vi "Project g.vi"() -> ()   [LabVIEW 2023]
uses:
  <vilib>/DAQmx/read.llb/DAQmx Read (Analog 1D DBL 1Chan NSamp).vi
  <vilib>/Analysis/baseanly.llb/Mean (DBL).vi
  <vilib>/DAQmx/create/channels.llb/DAQmx Create Channel (AI-Voltage-Basic).vi
  <vilib>/DAQmx/configure/timing.llb/DAQmx Timing (Sample Clock).vi
  <vilib>/DAQmx/configure/trigger.llb/DAQmx Start Trigger (Analog Edge).vi
  <vilib>/DAQmx/miscellaneous.llb/DAQmx Fill In Error Info.vi
  <vilib>/Analysis/NI_AALBase.lvlib
panel:
  in  "Elevation (m)":dbl
  in  "Latitude (rad)":dbl
  out "Experimental Acceleration (m/s²)":dbl
  out "Percent Error":dbl
  out "Theoretical Local Gravity Acceleration (m/s²)":dbl
  out "?":bool
  in  "File operation":T1(ring)=enum."open or create"
  in  "Select a file to save to":path
  out "Acceleration vs. Time":cluster{dbl[], "dX/dt":dbl[]}(graph)
  in  "Triggering system":bool
  in  "Sample mode":i32(ring)=10178 items=["Finite Samples"=10178, "Continuous Samples"=10123, "Hardware Timed Single Point"=12522]
  in  "# Samples":i32=1000
  in  "DAQ Rate":dbl=5000.0
  out "Displacement vs. Time":cluster{dbl[], dbl[]}(graph)
  in  "stop":bool
  in  "# Loops \n(For continuous samples)":i32
  in  "Custom scale name":tag="LaserDicplacement (mm)(ST06)(Monday)"
  in  "Physical channels":tag="cDAQ2Mod1/ai0"
  # "DAQ Input"
  # "File information"
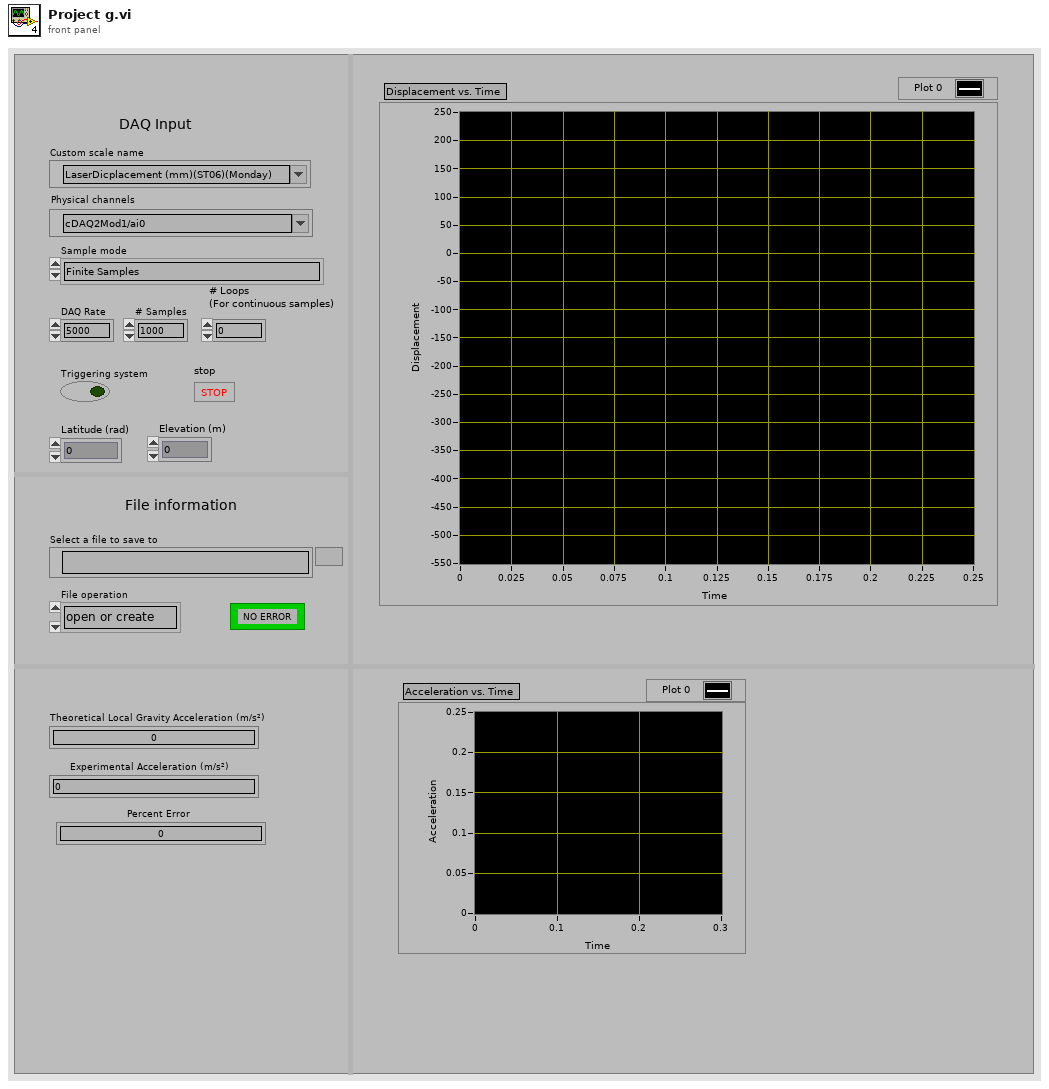
[diagram p1: front panel]
types:
  T1 = enum16{"open", "replace", "create", "open or create", "replace or create", "replace or create with confirmation"}
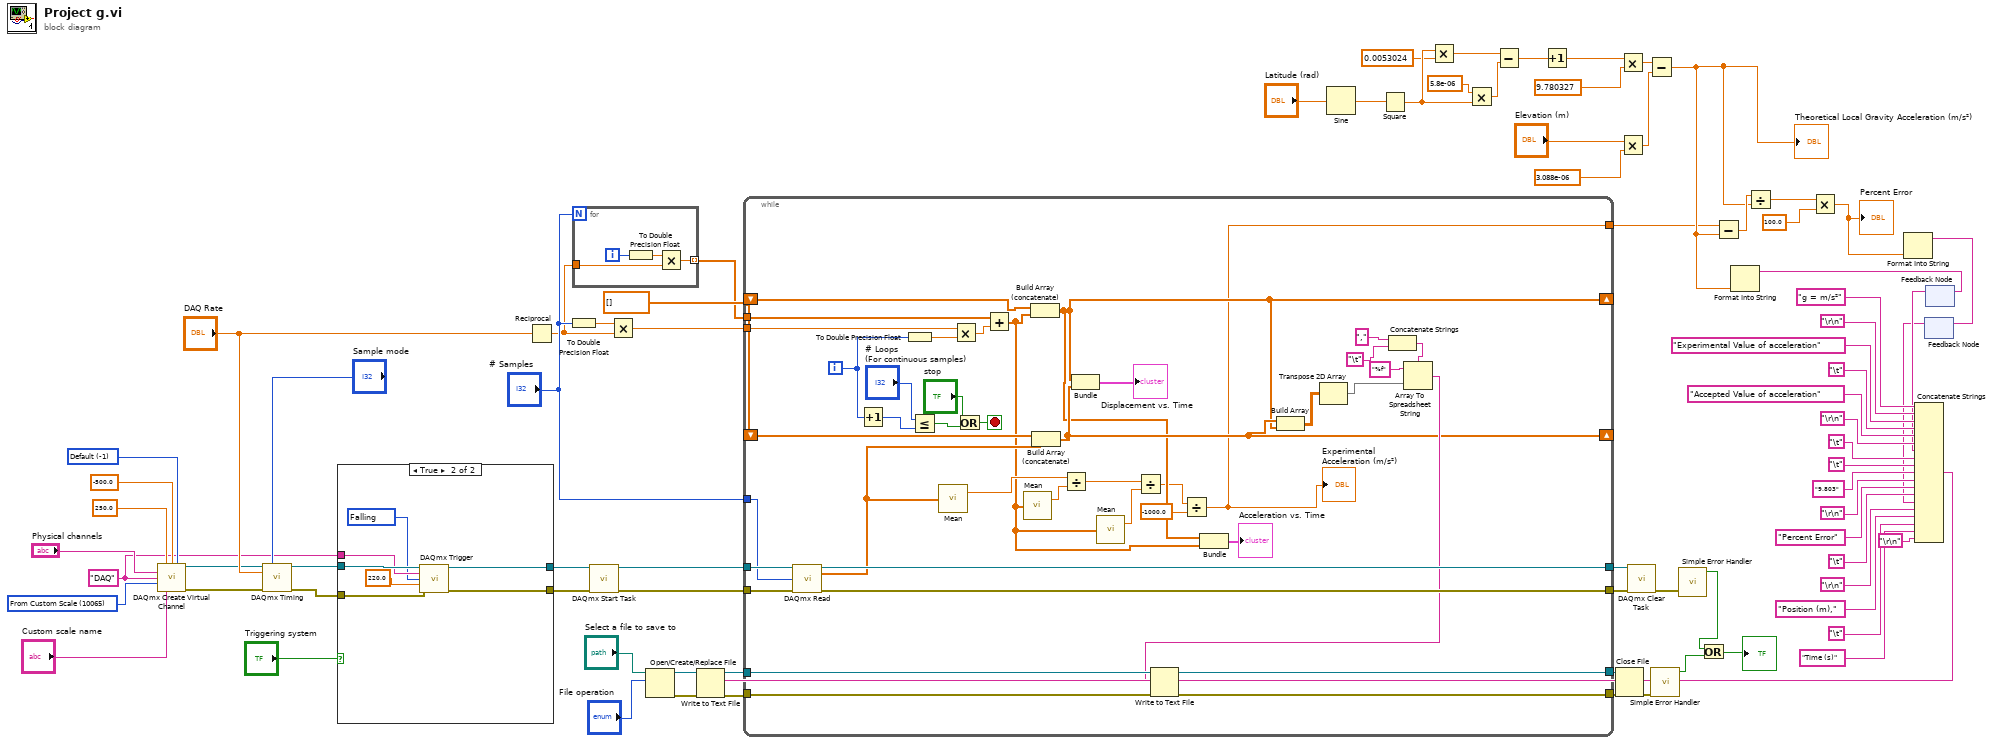
[diagram p0: block diagram]
diagram:
  w57 = "DAQ" ("name to assign")
  w71 = dbl[] []
  w76 = 10065 items=["Volts"=10348, "From Custom Scale"=10065] ("units")
  w79 = -1 items=["Default"=-1, "RSE"=10083, "NRSE"=10078, "Differential"=10106, "Pseudodifferential"=12529] ("input terminal configuration")
  n1 = call-poly <vilib>:"DAQmx Create Virtual Channel.vi"("maximum value"=250.0, "minimum value"=-500.0, "input terminal configuration"=w79, "physical channels"="Physical channels", "name to assign"=w57, "units"=w76, "custom scale name"="Custom scale name") -> ("task out"=w64:refnum<k21>, "error out"=w63:errorcluster)  [unwired: 7 in]
  n2 = call-poly <vilib>:"DAQmx Timing.vi"("task/channels in"=w64, "sample mode"="Sample mode", "rate"="DAQ Rate", "error in"=w63) -> ("task out"=w60:refnum<k21>, "error out"=w59:errorcluster)  [unwired: 10 in]
  n3 = case shown="True" "Triggering system" {
    tunnel: [w83 w86] -> w62
    tunnel: [w82 w85] -> w61
    tunnel: w60 -> [w83 w89]
    tunnel: w59 -> [w82 w88]
    tunnel: w57 -> [_ w87]
    frame False {
    }
    frame True {
      w84 = 10171 items=["Rising"=10280, "Falling"=10171] ("slope")
      n4 = call-poly <vilib>:"DAQmx Trigger.vi"("task/channels in"=w89, "source"=w87, "slope"=w84, "level"=220.0 ("window bottom"), "error in"=w88) -> ("task out"=w86:refnum<k21>, "error out"=w85:errorcluster)  [unwired: 9 in]
    }
  }
  n5 = Reciprocal(x="DAQ Rate") -> (1/x=w70:dbl)
  n6 = To Double Precision Float(number="# Samples") -> (double precision float=w73:dbl)
  n7 = for {
    N: "# Samples" -> [_]
    tunnel: w70 -> [w92]
    tunnel: [w91] -> w69 mode=indexing
    i -> [w94]
    n8 = To Double Precision Float(number=w94) -> (double precision float=w93:dbl)
    n9 = Multiply(x=w93, y=w92) -> (x*y=w91:dbl)
  }
  n10 = call <vilib>:"DAQmx Start Task.vi"("task/channels in"=w62, "error in"=w61) -> ("task out"=w67:refnum<k21>, "error out"=w66:errorcluster)  [unwired: 12 in]
  n11 = Multiply(x=w73, y=w70) -> (x*y=w72:dbl)
  n12 = Open/Create/Replace File(file path (use dialog)="Select a file to save to", operation (0:open)="File operation") -> (refnum out=w24:refnum<file>, error out=w23:errorcluster)  [unwired: 4 in, 1 out]
  n13 = Sine(x="Latitude (rad)") -> (sin(x)=w16:dbl)
  n14 = Square(x=w16) -> (x^2=w14:dbl)
  n15 = Multiply(x=w14, y=0.0053024) -> (x*y=w2:dbl)
  n16 = Multiply(x=5.8e-06, y=w14) -> (x*y=w3:dbl)
  n17 = Subtract(x=w2, y=w3) -> (x-y=w6:dbl)
  n18 = Increment(x=w6) -> (x+1=w7:dbl)
  n19 = Multiply(x=w7, y=9.780327) -> (x*y=w9:dbl)
  n20 = Multiply(x="Elevation (m)", y=3.088e-06) -> (x*y=w10:dbl)
  n21 = Subtract(x=w9, y=w10) -> (x-y=w5:dbl)
  "Theoretical Local Gravity Acceleration (m/s²)" <- w5
  n22 = Format Into String(w5) -> (resulting string=w21:string)  [unwired: 3 in, 1 out]
  n23 = feedback #1() -> (w20:string)  [unwired: 1 in]
  n24 = feedback #2() -> (w22:string)  [unwired: 1 in]
  n25 = Concatenate Strings("g = m/s²" ("string"), "\r\n", "Experimental Value of acceleration" ("string"), "\t", "Accepted Value of acceleration" ("string"), "\r\n", w22, "\t", "\t", "9.803" ("string"), "\r\n", "Percent Error" ("string"), "\t", w20, "\r\n", "Position (m),", "\t", "Time (s)", "\r\n") -> (w29:string)
  n26 = Write to Text File(file (use dialog)=w24, text=w29, error in=w23) -> (refnum out=w17:refnum<file>, error out=w18:errorcluster)  [unwired: 1 in, 1 out]
  n27 = while {
    shift-right: [w107] -> _
    shift-left: w71 -> [w126]
    shift-right: [w106] -> _
    shift-left: w71 -> [w105]
    tunnel: "# Samples" -> [w122]
    tunnel: w72 -> [w127]
    tunnel: w69 -> [w125]
    tunnel: w67 -> [w124]
    tunnel: w66 -> [w123]
    tunnel: [w120] -> w56
    tunnel: [w119] -> w55
    tunnel: [w118] -> w54
    tunnel: [w117] -> w53
    tunnel: w18 -> [w116]
    tunnel: w17 -> [w115]
    tunnel: [w95] -> w1
    i -> [w128]
    stop <- w132 stop-if-true
    n28 = call-poly <vilib>:"DAQmx Read.vi"("task/channels in"=w124, "number of samples per channel"=w122, "error in"=w123) -> ("task out"=w120:refnum<k21>, "data"=w102:dbl[], "error out"=w119:errorcluster)  [unwired: 10 in]
    n29 = Increment(x=w128) -> (x+1=w130:i32)
    n30 = To Double Precision Float(number=w128) -> (double precision float=w135:dbl)
    n31 = Less Or Equal?(x="# Loops \n(For continuous samples)", y=w130) -> (x <= y?=w129:bool)
    n32 = call-poly <vilib>:"Mean.vi"("X"=w102) -> ("mean"=w101:dbl)  [unwired: 1 out]
    n33 = Multiply(x=w127, y=w135) -> (x*y=w134:dbl)
    n34 = Or(x="stop", y=w129) -> (x .or. y?=w132:bool)
    n35 = Add(x=w125, y=w134) -> (x+y=w99:dbl[])
    n36 = call-poly <vilib>:"Mean.vi"("X"=w99) -> ("mean"=w98:dbl)  [unwired: 1 out]
    n37 = Build Array (concatenate)(w105, w99) -> (w106:dbl[])
    n38 = Build Array (concatenate)(w126, w102) -> (w107:dbl[])
    n39 = Divide(x=w101, y=w98) -> (x/y=w100:dbl)
    n40 = Bundle(w106, w107) -> (→"Displacement vs. Time":cluster{dbl[], dbl[]})  [unwired: 1 in]
    n41 = call-poly <vilib>:"Mean.vi"("X"=w99) -> ("mean"=w103:dbl)  [unwired: 1 out]
    n42 = Divide(x=w100, y=w103) -> (x/y=w96:dbl)
    n43 = Divide(x=w96, y=-1000.0) -> (x/y=w95:dbl)
    "Experimental Acceleration (m/s²)" <- w95
    n44 = Bundle(w106, w99) -> (→"Acceleration vs. Time":cluster{dbl[], dbl[]})  [unwired: 1 in]
    n45 = Build Array(w107, w106) -> (w112:dbl[][])
    n46 = Transpose 2D Array(2D array=w112) -> (transposed array=w111:dbl[][])
    n47 = Concatenate Strings("," ("delimiter (Tab)"), "\t") -> (w109:string)
    n48 = Array To Spreadsheet String(delimiter (Tab)=w109, array=w111, 3:"%f" ("format string")) -> (spreadsheet string=w113:string)
    n49 = Write to Text File(file (use dialog)=w115, text=w113, error in=w116) -> (refnum out=w118:refnum<file>, error out=w117:errorcluster)  [unwired: 1 in, 1 out]
  }
  n50 = Close File(refnum=w54, error in=w53) -> (error out=w50:errorcluster)  [unwired: 1 out]
  n51 = call <vilib>:"DAQmx Clear Task.vi"("task in"=w56, "error in"=w55) -> ("error out"=w78:errorcluster)  [unwired: 13 in]
  n52 = call <vilib>:"Simple Error Handler.vi"("error in (no error)"=w50) -> ("error?"=w49:bool)  [unwired: 4 in, 4 out]
  n53 = call <vilib>:"Simple Error Handler.vi"("error in (no error)"=w78) -> ("error?"=w48:bool)  [unwired: 4 in, 4 out]
  n54 = Or(x=w48, y=w49) -> (x .or. y?=→"?":bool)
  n55 = Subtract(x=w1, y=w5) -> (x-y=w28:dbl)
  n56 = Divide(x=w28, y=w5) -> (x/y=w27:dbl)
  n57 = Multiply(x=w27, y=100.0) -> (x*y=w25:dbl)
  "Percent Error" <- w25
  n58 = Format Into String(w25) -> (resulting string=w19:string)  [unwired: 3 in, 1 out]
  n59 = feedback-in #1(w19) -> ()
  n60 = feedback-in #2(w21) -> ()
